vi "workspace.free.vi"(8 "error in":errorcluster, 11 "Workspace in":refnum<class "Workspace.lvclass">) -> (0 "error out":errorcluster, 3 "Workspace out":refnum<class "Workspace.lvclass">)   [LabVIEW 2020, in "Workspace.lvclass"]
doc: "Releases the handle and its associated resources."
uses:
  Workspace.lvclass
  Workspace.lvclass/Workspace.ctl
  client.lvlib
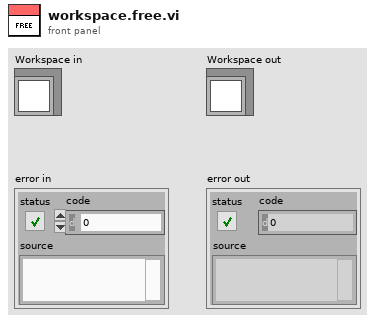
[diagram p1: front panel]
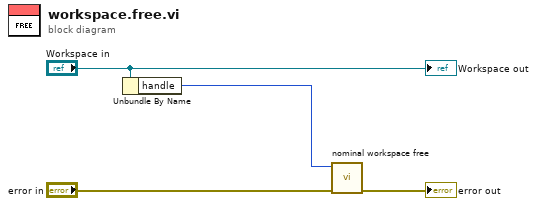
[diagram p0: block diagram]
diagram:
  n1 = Unbundle By Name("Workspace in") -> ("handle"=w2:i32)
  n2 = call "nominal workspace free.vi"("error in (no error)"="error in", "workspace"=w2) -> ("error out"=→"error out":errorcluster)  [unwired: 8 in, 1 out]
  "Workspace out" <- "Workspace in"
